vi "DaemonServ.vi"() -> ()   [LabVIEW 2011, in "WaveFormGraph.xctl"]
uses:
  WaveFormGraph.xctl
  CursorPosQueueCluster.ctl
  F:/Program Files/National Instruments/LabVIEW 2011/resource/importtools/Common/Event/NISAST Event.lvclass
panel:
  in  "UsrEvent":refnum<class "NISAST Event.lvclass">
  in  "CusorPos":T1
  # "切勿修改这些控件的名称, 因为XCTL 的Init.vi中使用了控件名称来初始化控件值."
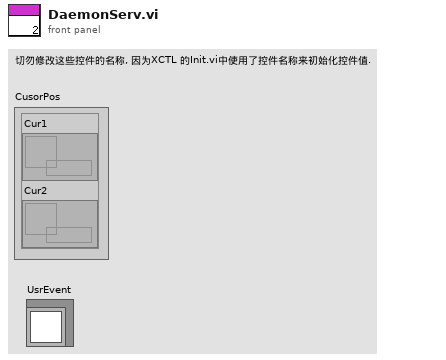
[diagram p1: front panel]
types:
  T1 = typedef "CursorPosQueueCluster.ctl" = cluster{"Cur1":refnum<queue>, "Cur2":refnum<queue>}
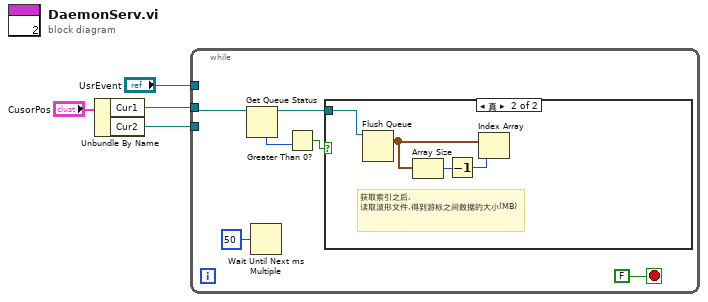
[diagram p0: block diagram]
diagram:
  n1 = Unbundle By Name("CusorPos") -> ("Cur1"=w2:refnum<queue>, "Cur2"=w1:refnum<queue>)
  n2 = while {
    tunnel: "UsrEvent" -> [_]
    tunnel: w2 -> [w10]
    tunnel: w1 -> [_]
    stop <- FALSE stop-if-true
    n3 = Get Queue Status(queue=w10) -> (queue out=w7:refnum<queue>, # elements in queue=w9:i32)  [unwired: 2 in, 6 out]
    n4 = Wait Until Next ms Multiple(millisecond multiple=u32 50 ("毫秒倍数")) -> ()  [unwired: 1 out]
    n5 = Greater Than 0?(x=w9) -> (x > 0?=w8:bool)
    n6 = case shown="真" w8 {
      tunnel: w7 -> [_ w14]
      frame False {
      }
      frame True {
        # "获取索引之后, 读取波形文件,得到游标之间数据的大小(MB)"
        n7 = Flush Queue(queue=w14) -> (remaining elements=w13:cluster{"X":dbl, "Y":dbl}[])  [unwired: 1 in, 2 out]
        n8 = Array Size(array=w13) -> (size(s)=w12:i32)
        n9 = Decrement(x=w12) -> (x-1=w11:i32)
        n10 = Index Array(array=w13, index=w11) -> ()  [unwired: 1 out]
      }
    }
  }
